vi "AO Continuous FPGA.vi"   [LabVIEW 2019]
uses:
  <vilib>/rvi/DataTransferAndStorage/Container/Common/niFpgaContainerGetUniqueNameForEmu.vi
  <vilib>/rvi/DataTransferAndStorage/Container/Common/niFpgaContainerSetEmuInfo.vi
  <vilib>/rvi/eio/common/nirviEmuReportErrorAndStop.vi
  <vilib>/rvi/LocalResourceManager/LocalResourceManager.xnode
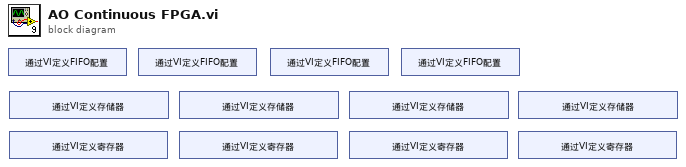
[diagram p0: block diagram]
diagram:
  n1 = xnode "通过VI定义FIFO配置"() -> ()  [unwired: 1 out]
  n2 = xnode "通过VI定义存储器"() -> ()  [unwired: 1 out]
  n3 = xnode "通过VI定义寄存器"() -> ()  [unwired: 1 out]
  n4 = xnode "通过VI定义FIFO配置"() -> ()  [unwired: 1 out]
  n5 = xnode "通过VI定义存储器"() -> ()  [unwired: 1 out]
  n6 = xnode "通过VI定义寄存器"() -> ()  [unwired: 1 out]
  n7 = xnode "通过VI定义FIFO配置"() -> ()  [unwired: 1 out]
  n8 = xnode "通过VI定义存储器"() -> ()  [unwired: 1 out]
  n9 = xnode "通过VI定义寄存器"() -> ()  [unwired: 1 out]
  n10 = xnode "通过VI定义FIFO配置"() -> ()  [unwired: 1 out]
  n11 = xnode "通过VI定义存储器"() -> ()  [unwired: 1 out]
  n12 = xnode "通过VI定义寄存器"() -> ()  [unwired: 1 out]
